vi "CreateWaveData.vi"(8 "error in (no error)":errorcluster, 11 "WaveGenerator in":refnum<class "WaveGenerator.lvclass">) -> (0 "error out":errorcluster, 2 "signal out":waveform(dbl), 3 "WaveGenerator out":refnum<class "WaveGenerator.lvclass">)   [LabVIEW 2021, in "WaveGenerator.lvclass"]
uses:
  WaveGenerator.lvclass
  C:/Program Files (x86)/National Instruments/LabVIEW 2021/vi.lib/addons/_Workers/Library/Classes/Worker/Worker.lvclass
  <vilib>/addons/_Workers/Library/Classes/Worker/Read ID.vi
  <vilib>/measure/NI_MABase.lvlib
  <vilib>/addons/_Workers/Library/Classes/Worker/Worker.lvclass
  C:/Program Files (x86)/National Instruments/LabVIEW 2021/vi.lib/addons/_Workers/Library/Classes/Workers Object/Workers Object.lvclass
  C:/Users/chrismadlax/Desktop/LVSampleCode/WorkersComposite/Workers/WaveGenerator/WaveGenerator.lvclass
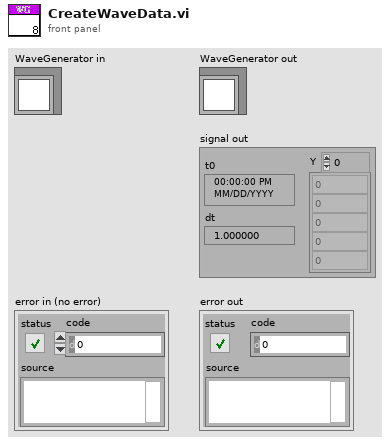
[diagram p1: front panel]
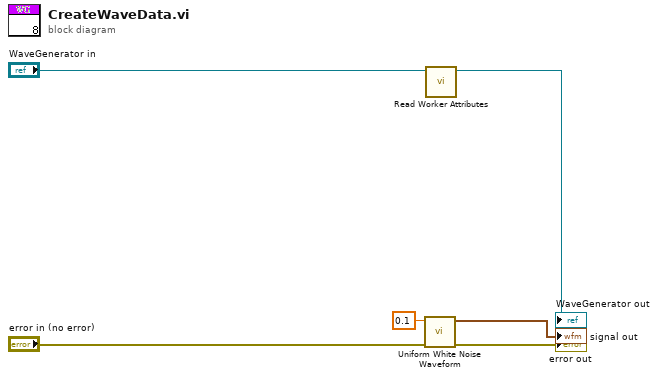
[diagram p0: block diagram]
diagram:
  n1 = call <vilib>:"Uniform White Noise Waveform.vi"("error in (no error)"="error in (no error)", "amplitude"=0.1 ("frequency")) -> ("error out"=→"error out":errorcluster, "signal out"=→"signal out":waveform(dbl))  [unwired: 8 in]
  n2 = call-poly <vilib>:"Read Worker Attributes.vi"("Worker"="WaveGenerator in") -> ("dup Worker out"=→"WaveGenerator out":refnum<class "WaveGenerator.lvclass">)  [unwired: 9 in, 1 out]
